vi "create_settings_file.vi"() -> ()   [LabVIEW 2010, in "GenericComponent.lvclass"]
uses:
  GenericComponent.lvclass
panel:
  in  "create button":bool
  in  "component path":path
  # "Settings file creator"
  # "This VI creates a first settings file for a component. You will have to fill in actual values by hand."
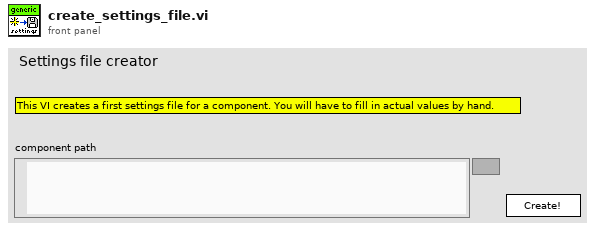
[diagram p1: front panel]
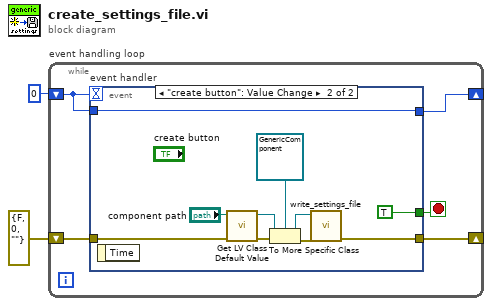
[diagram p0: block diagram]
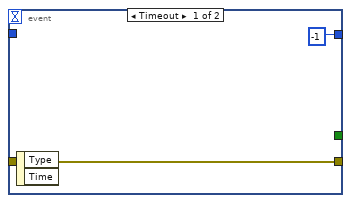
[diagram p2: hidden frame]
diagram:
  n1 = while "event handling loop" {
    shift-right: [w7] -> _
    shift-left: 0 -> [w6]
    shift-right: [w4] -> _
    shift-left: errorcluster {"status"=FALSE, "code"=0, "source"=""} ("error out") -> [w5]
    stop <- w3 stop-if-true
    n2 = event "event handler" shown="[1] \"create button\": Value Change" {
      selector: _ -> [_ _]
      dyn-events: _ -> [_ _]
      timeout: w6 -> [_ _]
      tunnel: [-1 w19] -> w7
      tunnel: w6 -> [_ w19]
      tunnel: w5 -> [w8 w18]
      tunnel: [w8 w16] -> w4
      tunnel: [_ TRUE] -> w3
      event Timeout {
        n3 = event-data() -> ()  [unwired: 1 in, 2 out]
      }
      event "create button": Value Change {
        n4 = event-data() -> ()  [unwired: 1 in, 1 out]
        n5 = call <vilib>:"Get LV Class Default Value.vi"("error in (no error)"=w18, "class path"="component path") -> ("error out"=w14:errorcluster, "object"=w13:refnum<class>)  [unwired: 8 in]
        n6 = To More Specific Class(target class=refnum<class "GenericComponent.lvclass"> refnum ("GenericPlugin.lvclass"), reference=w13, error in=w14) -> (specific class reference=w12:refnum<class "GenericComponent.lvclass">, error out=w15:errorcluster)
        n7 = call-dynamic "write_settings_file.vi"("error in (no error)"=w15, "GenericPlugin in"=w12) -> ("error out"=w16:errorcluster)  [unwired: 6 in, 3 out]
      }
    }
  }
